vi "Start Continuous Acquisition.vi"(0 "nSensorIP":u32, 1 "nMode":T1 items=["ACQ_INIT"=0, "DARK_MODE"=1, "BRIGHT_MODE"=2, "SOFTTRIGGER_MODE"=258, "SOFTTRIGGER_INSTANT_MODE"=259], 5 "refImg":u16[](array[numeric])=array[4097 elements], 7 "pImg":u16[](array[numeric])=array[4097 elements], 9 "nBuffLength":u32, 11 "error in (no error)":errorcluster, 12 "lpszRefPath":u8[](array[numeric])=array[4097 elements]) -> (4 "function return":i32, 6 "refImg out":u16[](array[numeric]), 8 "pImg out":u16[](array[numeric]), 15 "error out":errorcluster)   [LabVIEW 2022 SP3, in "BonTechDetector.lvlib"]
doc: "extern \"C\" BONTECHLIBRARY_API int __stdcall StartContinuousAcquisition(unsigned int nSensorIP, unsigned short* refImg, unsigned short* pImg, unsigned int nBuffLength, unsigned int nMode, LPCTSTR lpszRefPath);"
uses:
  BonTechDetector.lvlib
  Controls/Acquisition Commands.ctl
  Modules/Default Data/BonTechWrapperLibrary.dll
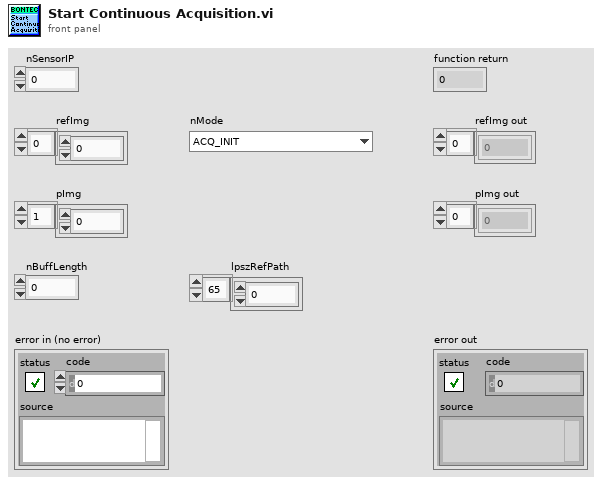
[diagram p1: front panel]
types:
  T1 = typedef "BonTechDetector.lvlib/Acquisition Commands.ctl" = u32
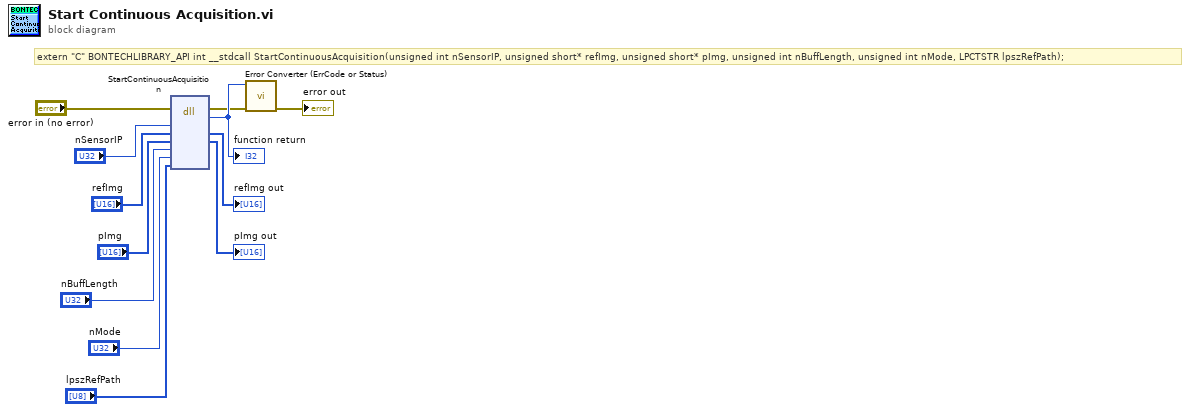
[diagram p0: block diagram]
diagram:
  # "extern \"C\" BONTECHLIBRARY_API int __stdcall StartContinuousAcquisition(unsigned int nSensorIP, unsigned short* refImg, unsigned short* pImg, unsigned int nBuffLength, unsigned int nMode, LPCTSTR lpszRefPath);"
  n1 = dll-call lib="E:/image-harvest/Modules/Default Data/BonTechWrapperLibrary.dll" fn="StartContinuousAcquisition"(error in="error in (no error)", "nSensorIP"="nSensorIP", "refImg"="refImg", "pImg"="pImg", "nBuffLength"="nBuffLength", "nMode"="nMode", "lpszRefPath"="lpszRefPath") -> (error out=w2:errorcluster, "return type"=w12:i32, "refImg"=→"refImg out":u16[], "pImg"=→"pImg out":u16[])  [unwired: 6 in, 1 out]
  "function return" <- w12
  n2 = call "Error Converter (ErrCode or Status).vi"("error in (no error)"=w2, "error code"=w12) -> ("error out"=→"error out":errorcluster)  [unwired: 9 in]
